vi "Index By HR.vi"(1 "Humidity Ratio [-]":dbl) -> (0 "HR Index":dbl)   [LabVIEW 2020]
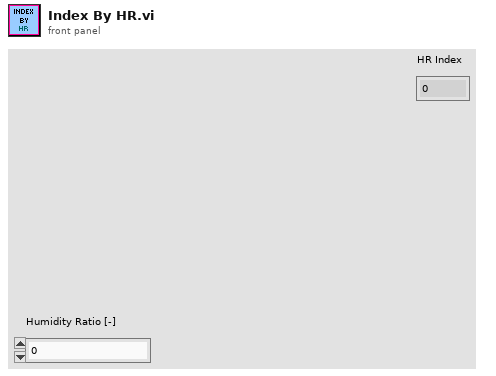
[diagram p1: front panel]
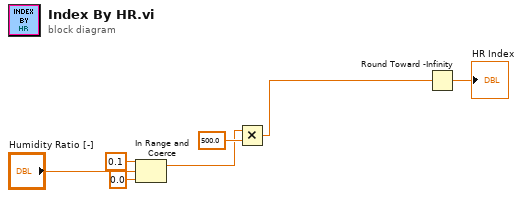
[diagram p0: block diagram]
diagram:
  n1 = In Range and Coerce(upper limit=0.1, x="Humidity Ratio [-]", lower limit=0.0) -> (coerced(x)=w4:dbl)  [unwired: 1 out]
  n2 = Multiply(x=w4, y=500.0) -> (x*y=w1:dbl)
  n3 = Round Toward -Infinity(1:w1) -> (0:→"HR Index":dbl)
